vi "classify error.vi"(8 "error to classify":errorcluster, 11 "Simple Sequencer TBM runtime in":refnum<class "Simple Sequencer TBM runtime.lvclass">) -> (0 "classified error":errorcluster, 2 "error classification":T1, 3 "Simple Sequencer TBM runtime out":refnum<class "Simple Sequencer TBM runtime.lvclass">)   [LabVIEW 2014, in "Simple Sequencer TBM runtime.lvclass"]
doc: "Allows a module to classify an error generated at any point during execution. This <b>error classification</b> can then be used by calling code to determine if execution can continue. In addition, this function can be used to allow a component to clear an error, convert an error to a warning, or attempt to recover from an error. Recovery may be attempted only if <b>attempt recovery?</b> is true."
uses:
  Simple Sequencer TBM runtime.lvclass
  <vilib>/NI/Tag Bus Module Framework/runtime/error classification.ctl
  <vilib>/NI/Tag Bus Module Framework/runtime/TBM module execution interface.lvclass
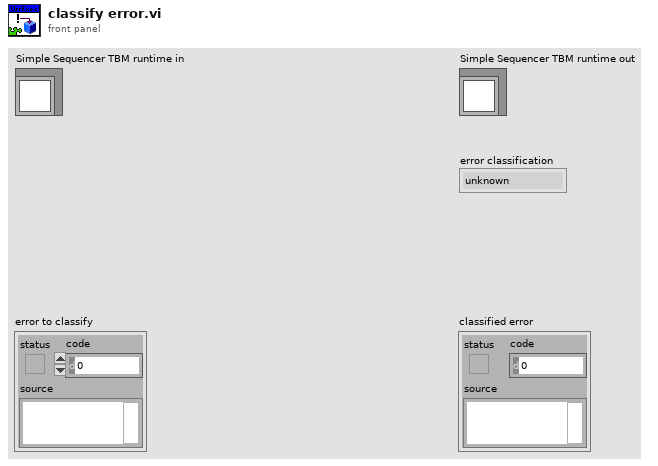
[diagram p1: front panel]
types:
  T1 = typedef "TBM module execution interface.lvclass/error classification.ctl" = enum16{"unknown", "none", "trivial", "recoverable", "critical"}
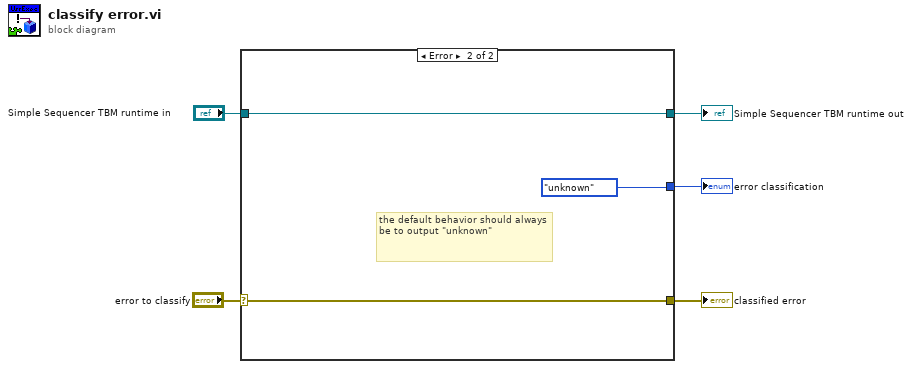
[diagram p0: block diagram]
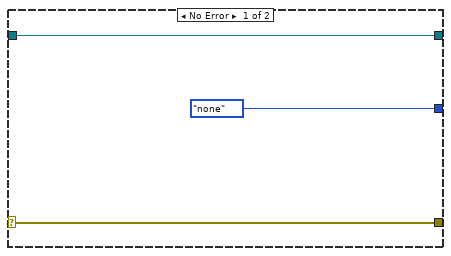
[diagram p2: hidden frame]
diagram:
  n1 = case shown="Error" "error to classify" {
    selector: "error to classify" -> [w7 w11]
    tunnel: [w8 w9] -> w4
    tunnel: "Simple Sequencer TBM runtime in" -> [w8 w9]
    tunnel: [w7 w11] -> w2
    tunnel: [error_classification."none" ("error classification") error_classification."unknown" ("error classification")] -> w1
    frame No Error {
    }
    frame Error {
      # "the default behavior should always be to output \"unknown\""
    }
  }
  "Simple Sequencer TBM runtime out" <- w4
  "error classification" <- w1
  "classified error" <- w2
